vi "Autonomous Independent.vi"() -> ()   [LabVIEW 2020]
doc: "This VI is called when autonomous begins, and will automatically be terminated when autonomous ends. You can carry out timed or sensor driven robot movement independently without needing to return to the caller."
uses:
  <vilib>/Rock Robotics/WPI/ThirdParty/JAS_Junk/TrajLib/PID_TUNING.ctl
  <vilib>/Rock Robotics/WPI/Utilities/WPI_GetSetVariantRefNum.vi
  Subsystems/Swerve/swerve_globals.vi
  <vilib>/addons/control/pid/NI_PID_pid.lvlib
  Subsystems/Magazine/magazine_globals.vi
  Subsystems/Shooter/shooter_globals.vi
  <vilib>/Rock Robotics/WPI/ThirdParty/JAS_Junk/TrajLib/Trajectory_Library.lvlib
  <vilib>/Rock Robotics/Network Tables/NT Read String.vi
  <vilib>/Rock Robotics/Network Tables/NT Write Numeric Array.vi
  <vilib>/addons/control/pid/pid.llb/PID (DBL).vi
panel:
  in  "XY PID Tuning":T1={"Kp"=5.0, "Ki"=0.001, "Kd"=0.0, "MaximumIntegral"=9.9e+30, "MinimumIntegral"=-9.9e+30}
  in  "Theta PID Tuning":T1={"Kp"=0.7, "Ki"=0.001, "Kd"=0.0, "MaximumIntegral"=9.9e+30, "MinimumIntegral"=-9.9e+30}
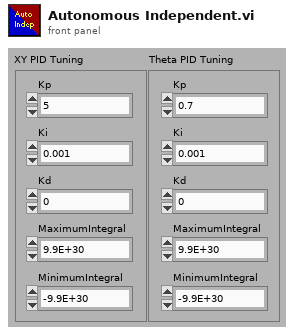
[diagram p1: front panel]
types:
  T1 = typedef "Trajectory_Library.lvlib/PID_TUNING.ctl" = cluster{"Kp":dbl, "Ki":dbl, "Kd":dbl, "MaximumIntegral":dbl, "MinimumIntegral":dbl}
  T2 = typedef "WPI_JoystickDevRef.ctl" = cluster{"Device":T3}
  T3 = typedef "WPI_JoystickDeviceEnum.ctl" = enum16{"USB 0", "USB 1", "USB 2", "USB 3", "USB 4", "USB 5"}
  T4 = cluster{"proportional gain (Kc)":dbl, "integral time (Ti, min)":dbl, "derivative time (Td, min)":dbl}
  T5 = typedef "CTRE_PigeonIMU_DeviceRef.ctl" = cluster{"DeviceStatus":errorcluster, "Device Number":u8, "Type":T6, "Device ID":u32, "Handle":u64, "UsageFrame":u32, "Library Path":path}
  T6 = typedef "CTRE_PigeonIMU_ConnectionType.ctl" = u32
  T7 = typedef "PathPlanner.lvlib/PathPlannerWaypoint.ctl" = cluster{"AnchorPoint":T8, "PrevControl":T8, "NextControl":T8, "HolonomicRotation":T9, "VelOverride":dbl, "isReversal":bool}
  T8 = typedef "Trajectory_Library.lvlib/TRANSLATION2D.ctl" = cluster{"X":dbl, "Y":dbl}
  T9 = typedef "Trajectory_Library.lvlib/ROTATION2D.ctl" = cluster{"VALUE":dbl, "COS":dbl, "SIN":dbl}
  T10 = typedef "Trajectory_Library.lvlib/HOLONOMIC_DRV_CTRL.ctl" = cluster{"poseTolerance":T11, "poseError":T11, "Enabled":bool, "PID_xCtrl":T12, "PID_yCtrl":T12, "PROF_PID_thetaCtrl":T13, "RotationError":T9, "FirstRun":bool}
  T11 = typedef "Trajectory_Library.lvlib/POSE2D.ctl" = cluster{"TRANSLATION":T8, "ROTATION":T9}
  T12 = typedef "Trajectory_Library.lvlib/PID_CONTROLLER.ctl" = cluster{"Kp":dbl, "Ki":dbl, "Kd":dbl, "Period":dbl, "Max_Integral":dbl, "Min_Integral":dbl, "Max_Input":dbl, "Min_Input":dbl, "Continuous":bool, "PositionError":dbl, "VelocityError":dbl, "PrevError":dbl, "TotalError":dbl, "PositionTolerance":dbl, "VelocityTolerance":dbl, "SetPoint":dbl, "Kf":dbl, "Prev_Deriv":dbl, "Prev_Deriv 2":dbl, "DerivativeFilter":bool, "Min_Output":dbl, "Max_Output":dbl, "Prev_F_P":dbl, "Prev_F_P_2":dbl, "AntiWindupActive":bool, "Measurement":dbl}
  T13 = typedef "Trajectory_Library.lvlib/PROFILED_PID_CONTROLLER.ctl" = cluster{"Controller":T12, "Goal":T14, "Setpoint":T14, "Constraint":T15}
  T14 = typedef "Trajectory_Library.lvlib/TRAPEZOID_PROFILE_STATE.ctl" = cluster{"Position":dbl, "Velocity":dbl}
  T15 = typedef "Trajectory_Library.lvlib/TRAPEZOID_PROFILE_CONSTRAINT.ctl" = cluster{"MaxVelocity":dbl, "MaxAcceleration":dbl}
  T16 = typedef "Trajectory_Library.lvlib/CHASSIS_SPEEDS.ctl" = cluster{"vX":dbl, "vY":dbl, "vOmega":dbl}
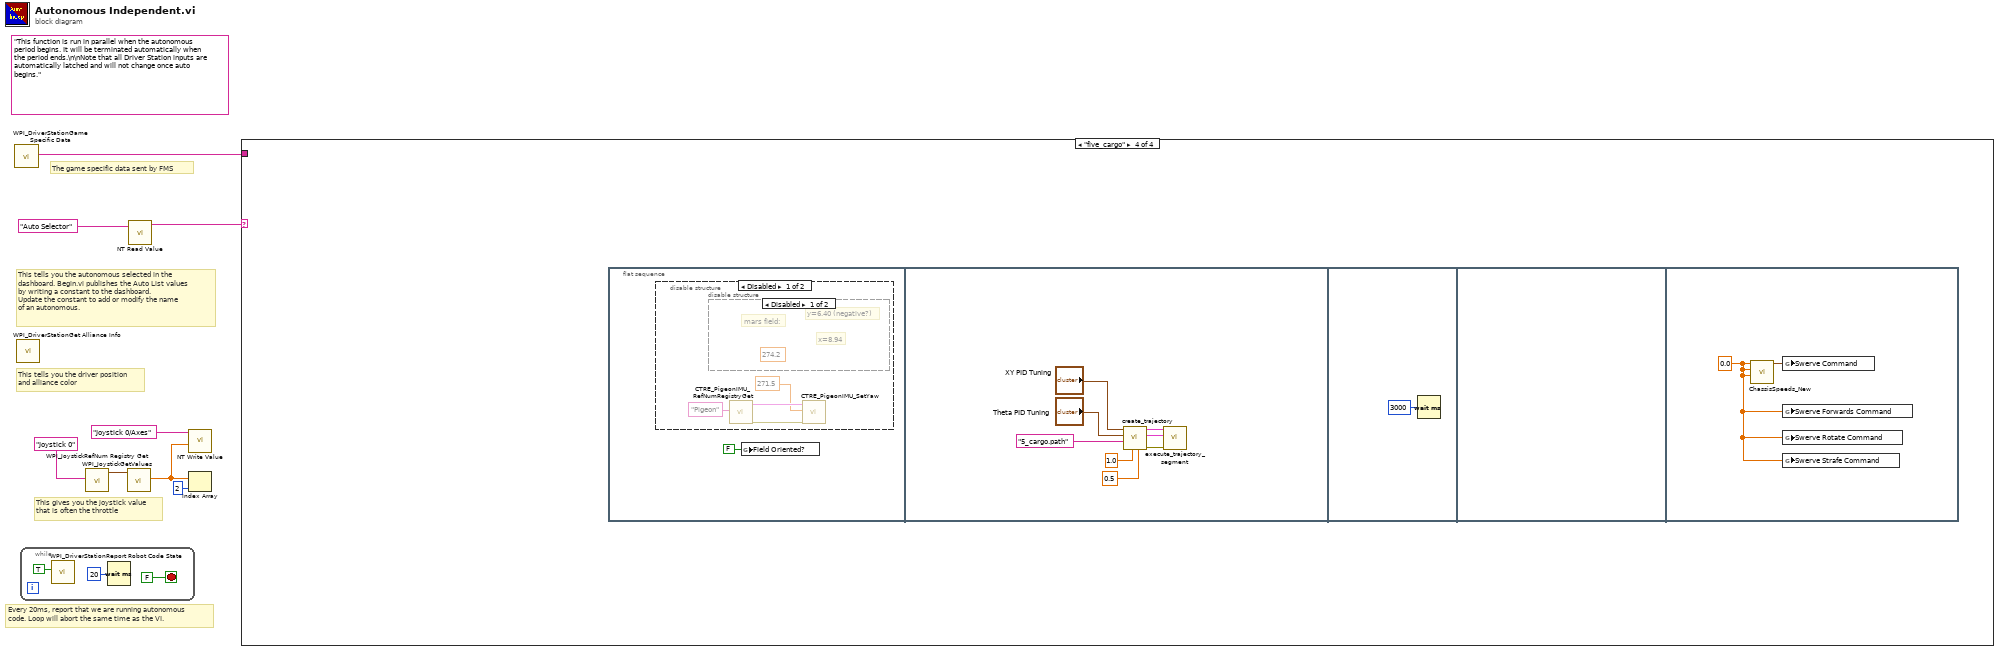
[diagram p0: block diagram]
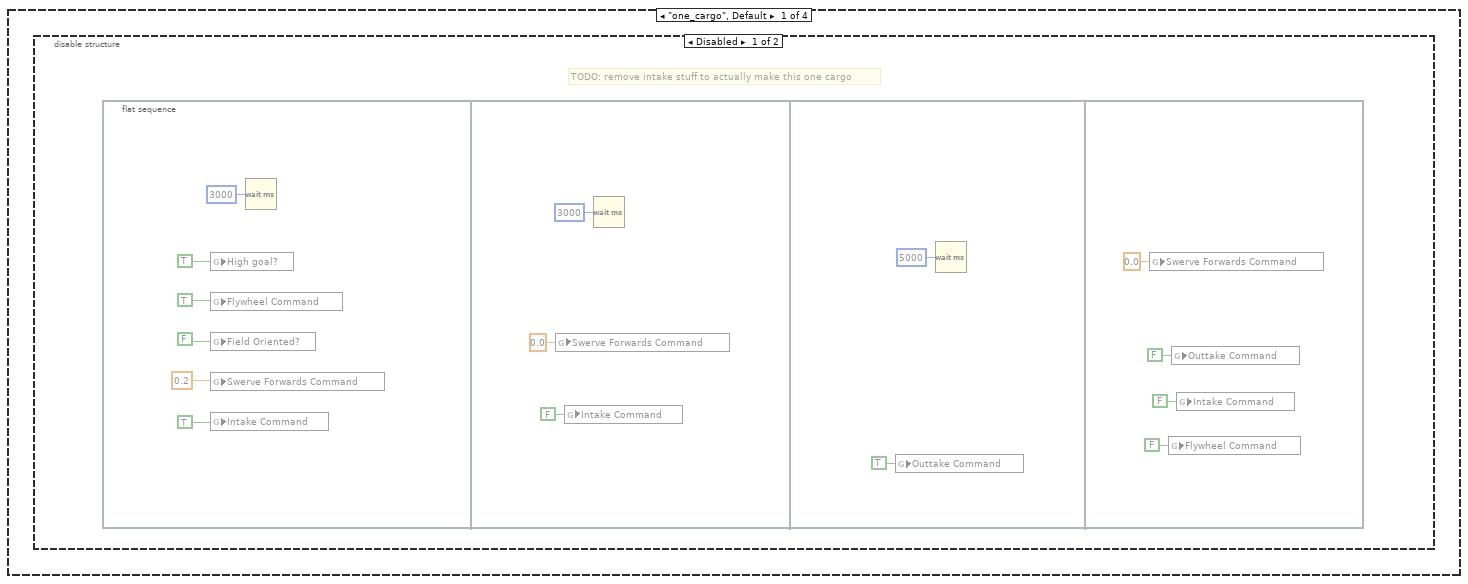
[diagram p2: hidden frame]
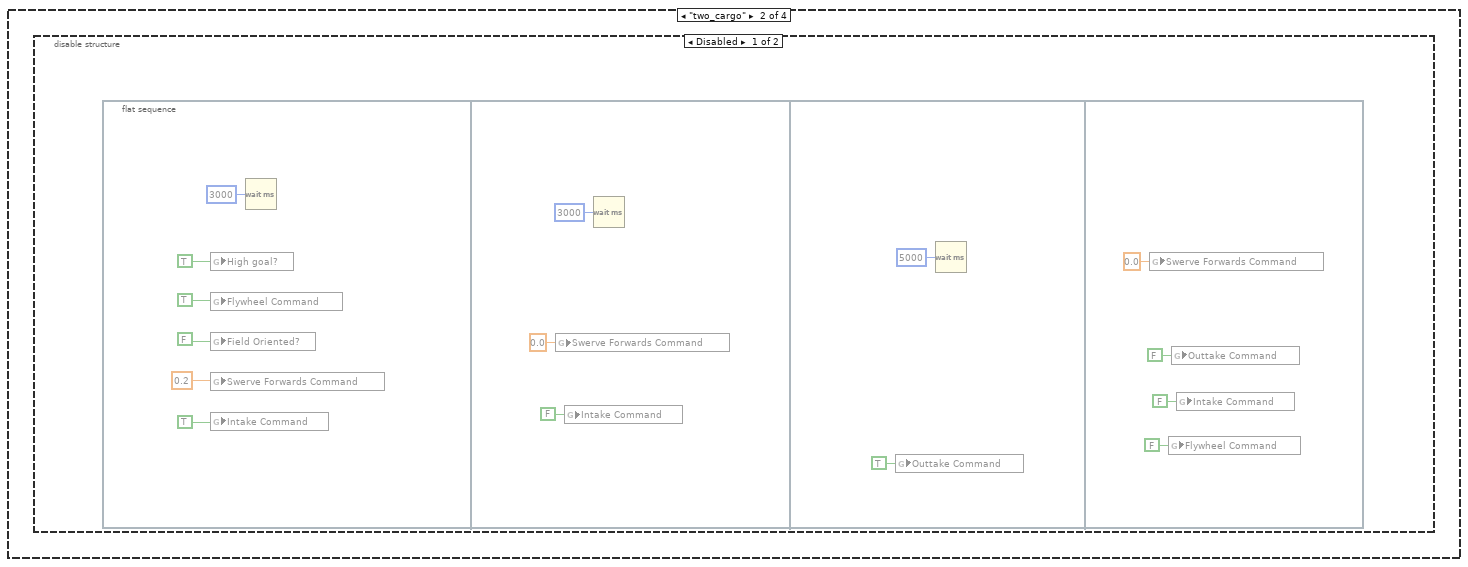
[diagram p4: hidden frame]
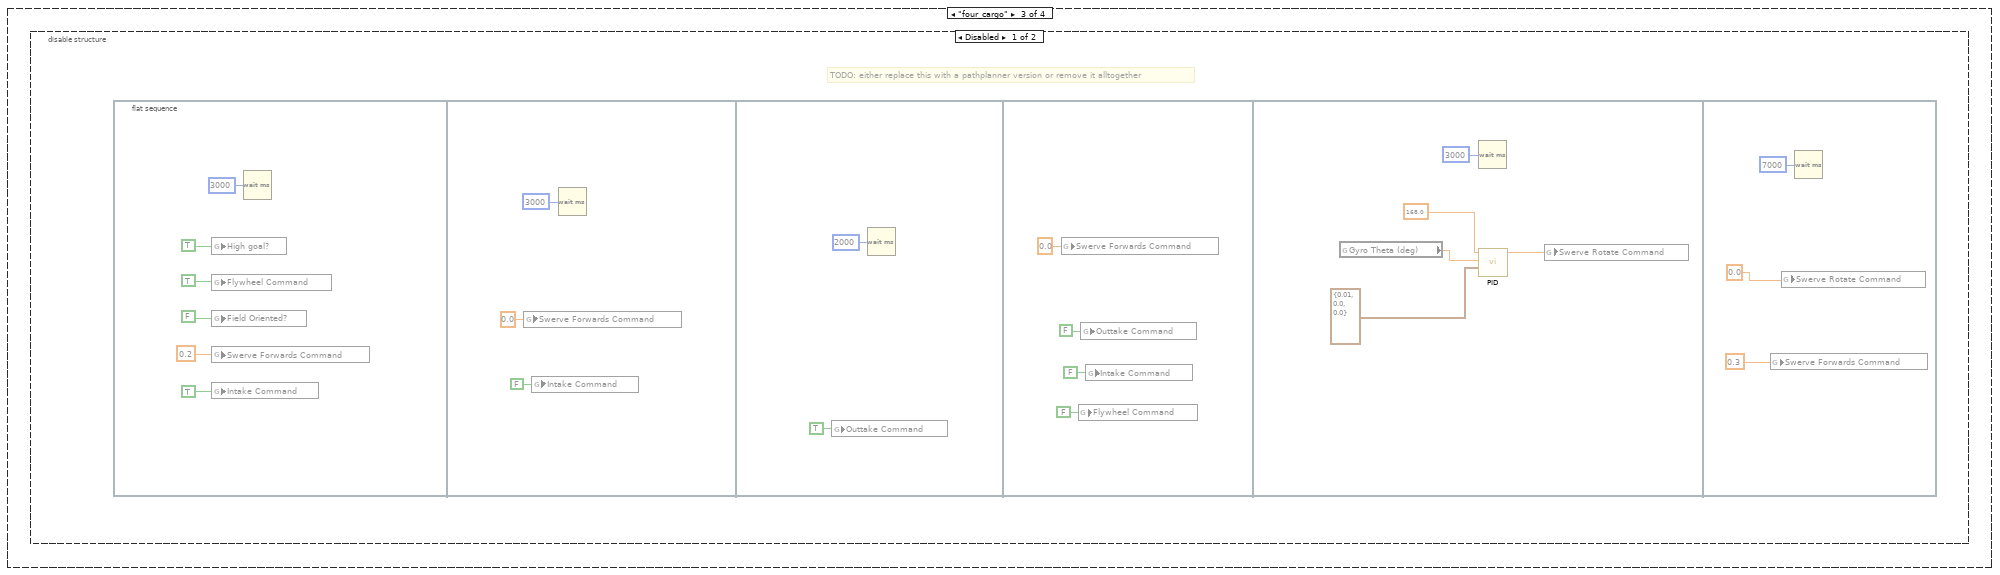
[diagram p6: hidden frame]
diagram:
  (unwired) "This function is run in parallel when the autonomous period begins. It will be terminated automatically when the period ends.\n\nNote that all Driver Station inputs are automatically latched and will not change once auto begins."
  # "The game specific data sent by FMS"
  # "This tells you the autonomous selected in the \ndashboard. Begin.vi publishes the Auto List values\nby writing a constant to the dashboard.\nUpdate the constant to add or modify the name\nof an autonomous."
  # "Every 20ms, report that we are running autonomous\ncode. Loop will abort the same time as the VI."
  # "This gives you the joystick value\nthat is often the throttle"
  # "This tells you the driver position\nand alliance color"
  n1 = call <vilib>:"WPI_DriverStationGame Specific Data.vi"() -> ("Game Specific Data"=w2:string)  [unwired: 11 in]
  n2 = call <vilib>:"WPI_DriverStationGet Alliance Info.vi"() -> ()  [unwired: 12 out]
  n3 = while {
    stop <- FALSE stop-if-true
    n4 = call <vilib>:"WPI_DriverStationReport Robot Code State.vi"("Autonomous"=TRUE) -> ()  [unwired: 10 in, 1 out]
    n5 = Wait (ms)(milliseconds to wait=u32 20) -> ()  [unwired: 1 out]
  }
  n6 = call <vilib>:"WPI_JoystickRefNum Registry Get.vi"("refnum name"="Joystick 0") -> ("JoystickDevRef"=w7:T2)  [unwired: 1 in, 9 out]
  n7 = call <vilib>:"WPI_JoystickGetValues.vi"("JoystickDevRef"=w7) -> ("Axes"=w4:dbl[])  [unwired: 6 in, 4 out]
  n8 = call-poly <vilib>:"NT Read Value.vi"("Name"="Auto Selector") -> ("String"=w1:string)  [unwired: 9 in, 1 out]
  n9 = call-poly <vilib>:"NT Write Value.vi"("Numeric Array"=w4, "Name"="Joystick 0/Axes") -> ()  [unwired: 9 in, 1 out]
  n10 = Index Array(array=w4, index=2) -> ()  [unwired: 1 out]
  n11 = case shown="\"five_cargo\"" w1 {
    tunnel: w2 -> [_ _ _ _]
    frame "one_cargo", Default {
      n12 = disable-structure shown="Disabled" {
        frame Disabled {
          # "TODO: remove intake stuff to actually make this one cargo"
          n13 = flat-sequence {
            frame #0 {
              n14 = global write "shooter_globals.vi" "High goal?"(TRUE ("Flywheel Command")) -> ()
              n15 = global write "shooter_globals.vi" "Flywheel Command"(TRUE ("Flywheel Command")) -> ()
              n16 = global write "swerve_globals.vi" "Field Oriented?"(FALSE ("Field Oriented?")) -> ()
              n17 = global write "swerve_globals.vi" "Swerve Forwards Command"(0.2 ("Swerve Forwards Command")) -> ()
              n18 = global write "magazine_globals.vi" "Intake Command"(TRUE ("Intake Command")) -> ()
              n19 = Wait (ms)(milliseconds to wait=u32 3000) -> ()  [unwired: 1 out]
            }
            frame #1 {
              n20 = global write "swerve_globals.vi" "Swerve Forwards Command"(0.0 ("Swerve Forwards Command")) -> ()
              n21 = global write "magazine_globals.vi" "Intake Command"(FALSE ("Intake Command")) -> ()
              n22 = Wait (ms)(milliseconds to wait=u32 3000) -> ()  [unwired: 1 out]
            }
            frame #2 {
              n23 = global write "magazine_globals.vi" "Outtake Command"(TRUE ("Outtake Command")) -> ()
              n24 = Wait (ms)(milliseconds to wait=u32 5000) -> ()  [unwired: 1 out]
            }
            frame #3 {
              n25 = global write "swerve_globals.vi" "Swerve Forwards Command"(0.0 ("Swerve Forwards Command")) -> ()
              n26 = global write "shooter_globals.vi" "Flywheel Command"(FALSE ("Flywheel Command")) -> ()
              n27 = global write "magazine_globals.vi" "Outtake Command"(FALSE ("Outtake Command")) -> ()
              n28 = global write "magazine_globals.vi" "Intake Command"(FALSE ("Intake Command")) -> ()
            }
          }
        }
        frame Enabled {
        }
      }
    }
    frame "two_cargo" {
      n29 = disable-structure shown="Disabled" {
        frame Disabled {
          n30 = flat-sequence {
            frame #0 {
              n31 = global write "shooter_globals.vi" "High goal?"(TRUE ("Flywheel Command")) -> ()
              n32 = global write "shooter_globals.vi" "Flywheel Command"(TRUE ("Flywheel Command")) -> ()
              n33 = global write "swerve_globals.vi" "Field Oriented?"(FALSE ("Field Oriented?")) -> ()
              n34 = global write "swerve_globals.vi" "Swerve Forwards Command"(0.2 ("Swerve Forwards Command")) -> ()
              n35 = global write "magazine_globals.vi" "Intake Command"(TRUE ("Intake Command")) -> ()
              n36 = Wait (ms)(milliseconds to wait=u32 3000) -> ()  [unwired: 1 out]
            }
            frame #1 {
              n37 = global write "swerve_globals.vi" "Swerve Forwards Command"(0.0 ("Swerve Forwards Command")) -> ()
              n38 = global write "magazine_globals.vi" "Intake Command"(FALSE ("Intake Command")) -> ()
              n39 = Wait (ms)(milliseconds to wait=u32 3000) -> ()  [unwired: 1 out]
            }
            frame #2 {
              n40 = global write "magazine_globals.vi" "Outtake Command"(TRUE ("Outtake Command")) -> ()
              n41 = Wait (ms)(milliseconds to wait=u32 5000) -> ()  [unwired: 1 out]
            }
            frame #3 {
              n42 = global write "swerve_globals.vi" "Swerve Forwards Command"(0.0 ("Swerve Forwards Command")) -> ()
              n43 = global write "shooter_globals.vi" "Flywheel Command"(FALSE ("Flywheel Command")) -> ()
              n44 = global write "magazine_globals.vi" "Outtake Command"(FALSE ("Outtake Command")) -> ()
              n45 = global write "magazine_globals.vi" "Intake Command"(FALSE ("Intake Command")) -> ()
            }
          }
        }
        frame Enabled {
        }
      }
    }
    frame "four_cargo" {
      n46 = disable-structure shown="Disabled" {
        frame Disabled {
          # "TODO: either replace this with a pathplanner version or remove it alltogether"
          n47 = flat-sequence {
            frame #0 {
              n48 = global write "shooter_globals.vi" "High goal?"(TRUE ("Flywheel Command")) -> ()
              n49 = global write "shooter_globals.vi" "Flywheel Command"(TRUE ("Flywheel Command")) -> ()
              n50 = global write "swerve_globals.vi" "Field Oriented?"(FALSE ("Field Oriented?")) -> ()
              n51 = global write "swerve_globals.vi" "Swerve Forwards Command"(0.2 ("Swerve Forwards Command")) -> ()
              n52 = global write "magazine_globals.vi" "Intake Command"(TRUE ("Intake Command")) -> ()
              n53 = Wait (ms)(milliseconds to wait=u32 3000) -> ()  [unwired: 1 out]
            }
            frame #1 {
              n54 = global write "swerve_globals.vi" "Swerve Forwards Command"(0.0 ("Swerve Forwards Command")) -> ()
              n55 = global write "magazine_globals.vi" "Intake Command"(FALSE ("Intake Command")) -> ()
              n56 = Wait (ms)(milliseconds to wait=u32 3000) -> ()  [unwired: 1 out]
            }
            frame #2 {
              n57 = global write "magazine_globals.vi" "Outtake Command"(TRUE ("Outtake Command")) -> ()
              n58 = Wait (ms)(milliseconds to wait=u32 2000) -> ()  [unwired: 1 out]
            }
            frame #3 {
              n59 = global write "swerve_globals.vi" "Swerve Forwards Command"(0.0 ("Swerve Forwards Command")) -> ()
              n60 = global write "shooter_globals.vi" "Flywheel Command"(FALSE ("Flywheel Command")) -> ()
              n61 = global write "magazine_globals.vi" "Outtake Command"(FALSE ("Outtake Command")) -> ()
              n62 = global write "magazine_globals.vi" "Intake Command"(FALSE ("Intake Command")) -> ()
            }
            frame #4 {
              n63 = global read "swerve_globals.vi" "Gyro Theta (deg)"() -> (w59:dbl)
              n64 = Wait (ms)(milliseconds to wait=u32 3000) -> ()  [unwired: 1 out]
              n65 = call-poly <vilib>:"PID.vi"("PID gains"=T4 {"proportional gain (Kc)"=0.01, "integral time (Ti, min)"=0.0, "derivative time (Td, min)"=0.0}, "process variable"=w59, "setpoint"=168.0 ("process variable")) -> ("output"=w57:dbl)  [unwired: 7 in, 1 out]
              n66 = global write "swerve_globals.vi" "Swerve Rotate Command"(w57) -> ()
            }
            frame #5 {
              n67 = global write "swerve_globals.vi" "Swerve Forwards Command"(0.3 ("Swerve Forwards Command")) -> ()
              n68 = global write "swerve_globals.vi" "Swerve Rotate Command"(0.0 ("Swerve Rotate Command")) -> ()
              n69 = Wait (ms)(milliseconds to wait=u32 7000) -> ()  [unwired: 1 out]
            }
          }
        }
        frame Enabled {
        }
      }
    }
    frame "five_cargo" {
      n70 = flat-sequence {
        frame #0 {
          n71 = disable-structure shown="Disabled" {
            frame Disabled {
              n72 = disable-structure shown="Disabled" {
                frame Disabled {
                  (unwired) 274.2 ("Value")
                  # "y=6.40 (negative?)"
                  # "x=8.94"
                  # "mars field:"
                }
                frame Enabled {
                }
              }
              n73 = call <vilib>:"CTRE_PigeonIMU_RefNumRegistryGet.vi"("refnum name"="Pigeon") -> ("error out"=w67:errorcluster, "PigeonIMUDevRef"=w68:T5)  [unwired: 9 in]
              n74 = call <vilib>:"CTRE_PigeonIMU_SetYaw.vi"("error in (no error)"=w67, "Value"=271.5, "PigeonIMUDevRef"=w68) -> ()  [unwired: 7 in, 2 out]
            }
            frame Enabled {
            }
          }
          n75 = global write "swerve_globals.vi" "Field Oriented?"(FALSE ("Field Oriented?")) -> ()
        }
        frame #1 {
          n76 = call "create_trajectory.vi"("Theta Max Accel"=0.5, "Theta Max Speed"=1.0, "File Name"="5_cargo.path", "Theta PID Tuning"="Theta PID Tuning", "XY PID Tuning"="XY PID Tuning") -> ("error out"=w72:errorcluster, "PathPlannerWayPoints"=w73:T7[], "outHOLONOMIC_DRV_CTRL"=w74:T10)  [unwired: 4 in]
          n77 = call "execute_trajectory_segment.vi"("error in"=w72, "in PathPlannerWayPoints"=w73, "inHOLONOMIC_DRV_CTRL"=w74) -> ()  [unwired: 6 in, 3 out]
        }
        frame #2 {
          n78 = Wait (ms)(milliseconds to wait=u32 3000) -> ()  [unwired: 1 out]
        }
        frame #3 {
        }
        frame #4 {
          w79 = 0.0 ("vX")
          n79 = call <vilib>:"ChassisSpeeds_New.vi"("vAngular"=w79, "vY"=w79, "vX"=w79) -> ("CHASSIS"=w80:T16)  [unwired: 8 in]
          n80 = global write "swerve_globals.vi" "Swerve Command"(w80) -> ()
          n81 = global write "swerve_globals.vi" "Swerve Forwards Command"(w79) -> ()
          n82 = global write "swerve_globals.vi" "Swerve Rotate Command"(w79) -> ()
          n83 = global write "swerve_globals.vi" "Swerve Strafe Command"(w79) -> ()
        }
      }
    }
  }
